vi "Write.vi"(0 "UdsHandleIn":T1={"LogPath"=path "", "LogEnabled"=FALSE, "isOpen"=FALSE, "LogContent"="", "Adapter"="CAN0", "MCanHandle"={"MCanAdapter"=refnum}, "TransmittId"=0, "ReceiveId"=0}, 1 "Frame":string="031 3C 00 00 00 00 00 00 0A", 3 "error in":errorcluster, 5 "LogSuspend":bool) -> (7 "UdsHandleOut":T1={"LogPath"=path "", "LogEnabled"=FALSE, "isOpen"=FALSE, "LogContent"="", "Adapter"="CAN0", "MCanHandle"={"MCanAdapter"=refnum}, "TransmittId"=0, "ReceiveId"=0}, 10 "error out":errorcluster)   [LabVIEW 2011, in "Konvolucio MUDS150628.lvlib"]
uses:
  <instrlib>/Konvolucio MUDS150628/Konvolucio MUDS150628.lvlib
  <instrlib>/Konvolucio MUDS150628/Types/UdsHandleType.ctl
  <instrlib>/Konvolucio MCAN120803/Types/MCanHandleType.ctl
  C:/Program Files/National Instruments/LabVIEW 2011/instr.lib/Konvolucio MCAN120803/Private/Konvolucio.MCAN120803.dll
  Konvolucio MCAN120803/Private/Konvolucio.MCAN120803.dll
  <instrlib>/Konvolucio MUDS150628/Private/UdsLogCanTxMessage.vi
  <instrlib>/Konvolucio MCAN120803/Konvolucio MCAN120803.lvlib
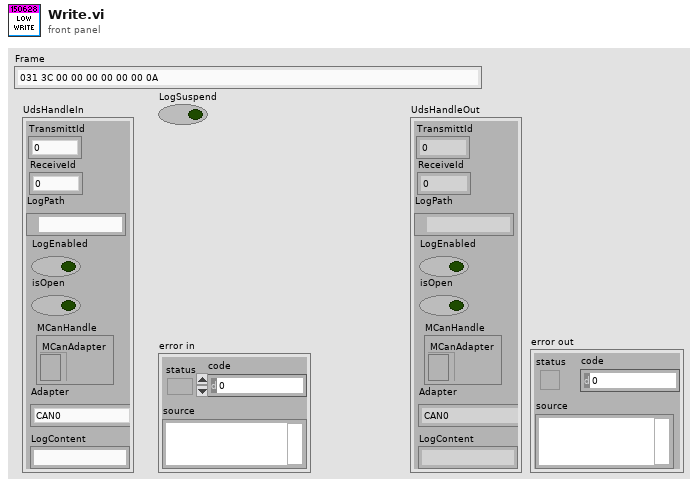
[diagram p1: front panel]
types:
  T1 = typedef "Konvolucio MUDS150628.lvlib/UdsHandleType.ctl" = cluster{"LogPath":path, "LogEnabled":bool, "isOpen":bool, "LogContent":string, "Adapter":string, "MCanHandle":T2, "TransmittId":u32, "ReceiveId":u32}
  T2 = typedef "Konvolucio MCAN120803.lvlib/MCanHandleType.ctl" = cluster{"MCanAdapter":refnum<k24>}
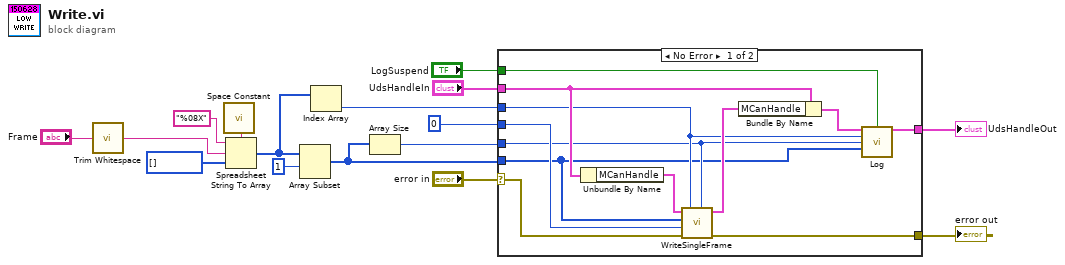
[diagram p0: block diagram]
diagram:
  n1 = call <vilib>:"Trim Whitespace.vi"("string"="Frame") -> ("trimmed string"=w6:string)  [unwired: 1 in]
  n2 = call <vilib>:"Space Constant.vi"() -> ("String"=w7:string)
  n3 = Spreadsheet String To Array(delimiter (Tab)=w7, format string="%08X", spreadsheet string=w6, array type (2D Dbl)=u32[] [] ("Response")) -> (array=w11:u32[])
  n4 = Array Subset(array=w11, index=1) -> (w2:u32[])  [unwired: 1 in]
  n5 = Index Array(array=w11) -> (element=w4:u32)  [unwired: 1 in]
  n6 = Array Size(array=w2) -> (size(s)=w3:i32)
  n7 = case shown="No Error" "error in" {
    selector: "error in" -> [w24 w29]
    tunnel: "LogSuspend" -> [w18 _]
    tunnel: "UdsHandleIn" -> [w23 w30]
    tunnel: [w26 w29] -> w14
    tunnel: [w17 w30] -> w13
    tunnel: w4 -> [w21 _]
    tunnel: w3 -> [w20 _]
    tunnel: w2 -> [w19 _]
    tunnel: u8 0 ("IsRemote") -> [w27 _]
    frame No Error {
      n8 = Unbundle By Name(w23) -> ("MCanHandle"=w28:T2)
      n9 = call <instrlib>:"WriteSingleFrame.vi"("ArbitrationId"=w21, "DataLength"=w20, "error in"=w24, "IsRemote"=w27, "Data"=w19, "MCanHandleIn"=w28) -> ("error out"=w26:errorcluster, "MCanHandleOut"=w25:T2)  [unwired: 4 in]
      n10 = Bundle By Name(cluster=w23, "MCanHandle"=w25) -> (w22:T1)
      n11 = call-poly <instrlib>:"Log.vi"("UdsHandleIn"=w22, "LogSuspend"=w18, "Id"=w21, "DataLength"=w20, "Data"=w19) -> ("UdsHandleOut"=w17:T1)  [unwired: 9 in, 1 out]
    }
    frame Error {
    }
  }
  "error out" <- w14
  "UdsHandleOut" <- w13
